vi "CFU_5p2_UCweesesr.vi"() -> ()   [LabVIEW 2016]
uses:
  <vilib>/express/express arith-compare/Formula/XNode/ExpressFormulaBlockNode.xnode
panel:
  out "Critically Dampened":string
  out "Over Dampened":string
  out "Underdampened":string
  in  "K":dbl
  in  "C":dbl
  in  "M":dbl
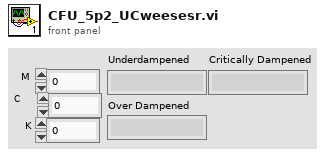
[diagram p1: front panel]
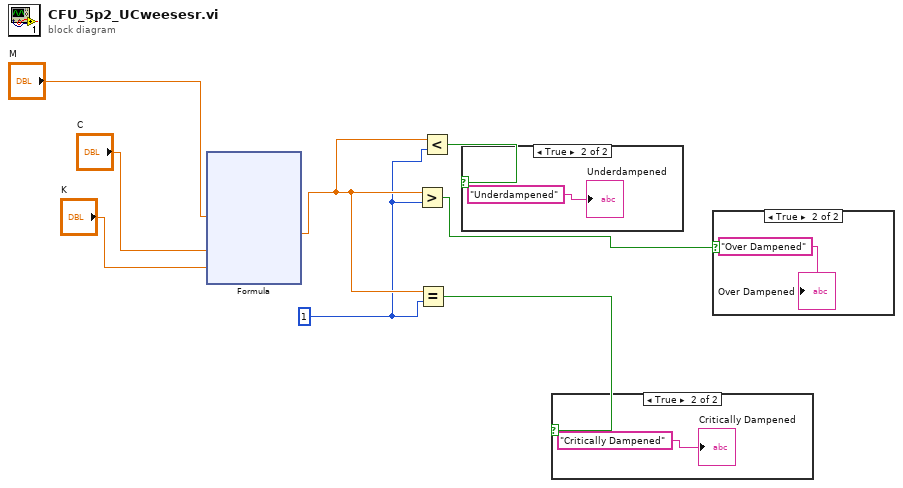
[diagram p0: block diagram]
diagram:
  w4 = 1
  n1 = xnode "Formula"("M"="M", "C"="C", "K"="K") -> ("Result"=w5:dbl)  [unwired: 1 in, 1 out]
  n2 = Greater?(x=w5, y=w4) -> (0:w2:bool)
  n3 = Equal?(x=w5, y=w4) -> (x = y?=w1:bool)
  n4 = Less?(x=w5, y=w4) -> (x < y?=w3:bool)
  n5 = case shown="True" w3 {
    frame False {
    }
    frame True {
      "Underdampened" <- "Underdampened"
    }
  }
  n6 = case shown="True" w1 {
    frame False {
    }
    frame True {
      "Critically Dampened" <- "Critically Dampened"
    }
  }
  n7 = case shown="True" w2 {
    frame False {
    }
    frame True {
      "Over Dampened" <- "Over Dampened"
    }
  }
